vi "IntelligentServo.vi"(2 "timeout (s) 2":dbl=10.0 caption="ONTime" format="%0.2f", 3 "number of samples":i32=30, 4 "timeout (s)":dbl=10.0 format="%0.2f", 5 "error in":errorcluster, 7 "stop (T)":bool=TRUE, 10 "device name":tag="myDAQ1") -> (14 "task out":refnum<k21>, 19 "error out":errorcluster)   [LabVIEW 2023]
doc: "Creates, edits, and runs tasks using NI-DAQmx. Refer to the NI-DAQmx Readme for a complete listing of devices NI-DAQmx supports.\n\nWhen you place this Express VI on the block diagram, the DAQ Assistant launches to create a new task. After you create a task, you can double-click the DAQ Assistant Express VI to edit that task. For continuous measurement or generation, place a while loop around the DAQ Assistant Express VI.\n\nUsing the DAQ Assistant Express VI creates a task accessible only to the Express VI. To make the task globally accessible from any application, you must convert the Express VI to an NI-DAQmx task saved in MAX\n\nYou can generate NI-DAQmx API code from a DAQ Assistant Express VI. Right-click the DAQ Assistant Express VI and select <B> Generate NI-DAQmx Code</B> from the shortcut menu to generate both configuration and example code for the task.\n\nFor continuous single-point input or output, the DAQ Assistant Express VI might not provide optimal performance. Refer to the Cont Acq&Graph Voltage-Single Point Optimization VI in examples\\DAQmx\\Analog In\\Measure Voltage.llb for an example of techniques to create higher-performance, single-point I/O applications."
uses:
  <vilib>/DAQmx/create/channels.llb/DAQmx Create Channel (CO-Pulse Generation-Time).vi
  <vilib>/DAQmx/configure/timing.llb/DAQmx Timing (Implicit).vi
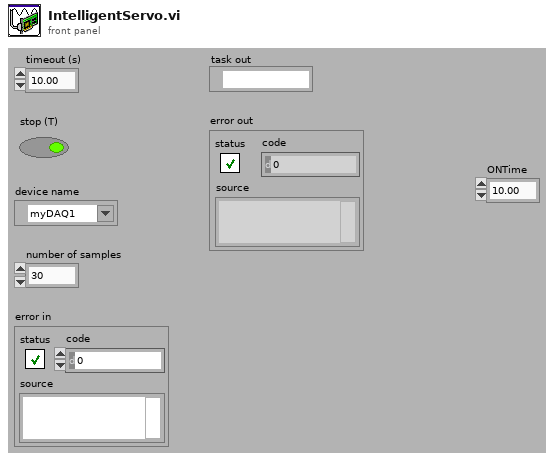
[diagram p1: front panel]
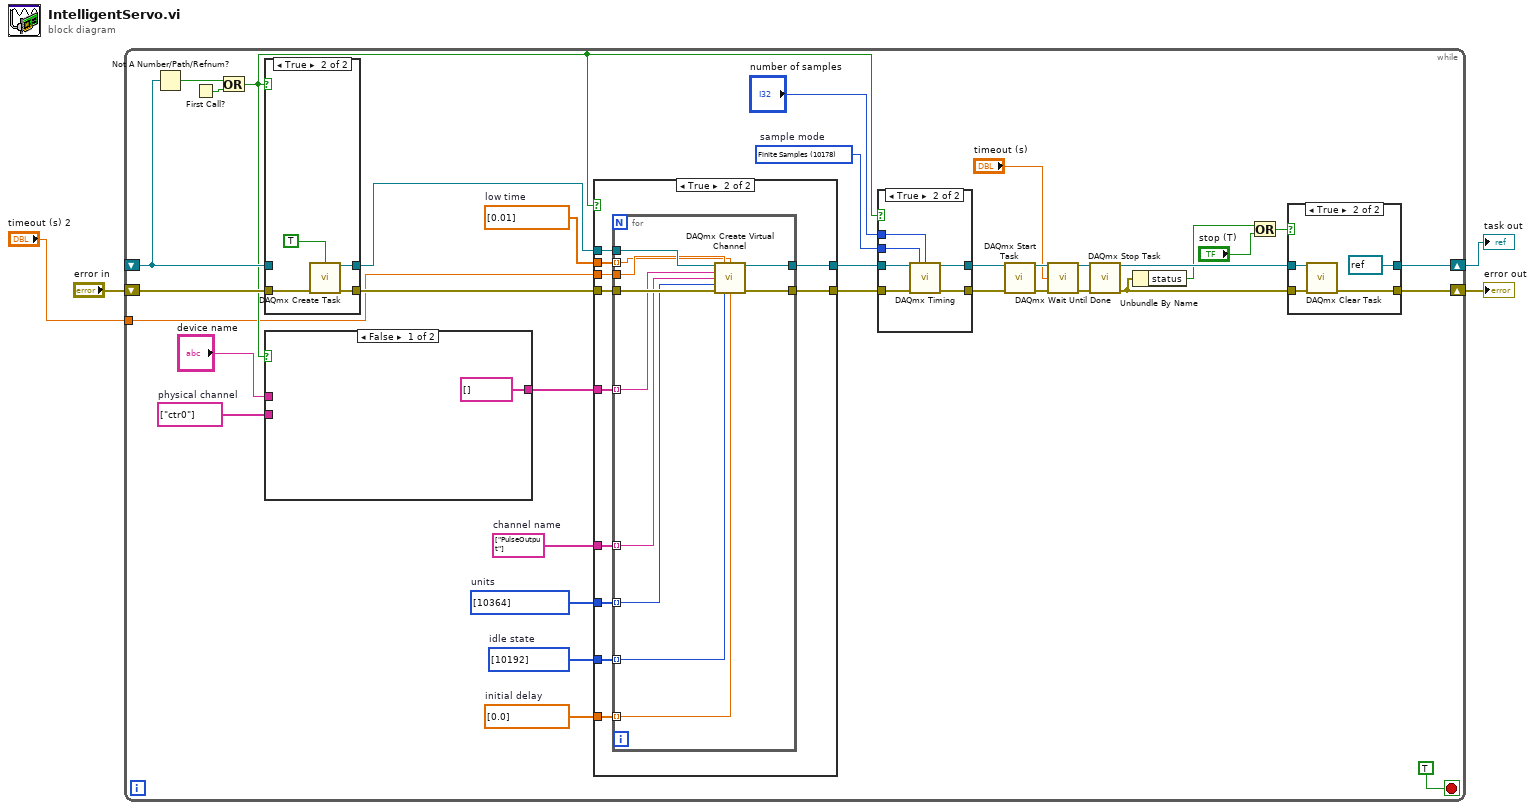
[diagram p0: block diagram]
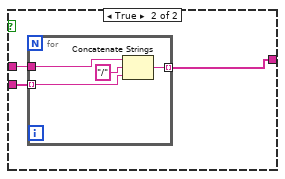
[diagram p5: hidden frame]
diagram:
  n1 = while {
    shift-right: [w12] -> w2
    shift-left: _ -> [w36]
    shift-right: [w6] -> w3
    shift-left: "error in" -> [w37]
    tunnel: "timeout (s) 2" -> [w5]
    stop <- TRUE stop-if-true
    w20 = 10178 items=["Finite Samples"=10178, "Continuous Samples"=10123, "Hardware Timed Single Point"=12522]  # sample mode
    w25 = dbl[] [0.0]  # initial delay
    w26 = i32[] [10192] items=["High"=10192, "Low"=10214]  # idle state
    w27 = i32[] [10364] items=["Seconds"=10364, "From Custom Scale"=10065]  # units
    w28 = string[] ["PulseOutput"]  # channel name
    w30 = dbl[] [0.01]  # low time
    w33 = string[] ["ctr0"]  # physical channel
    n2 = Not A Number/Path/Refnum?(number/path/refnum=w36) -> (NaN/Path/Refnum?=w35:bool)
    n3 = First Call?() -> (First Call?: T/F=w38:bool)
    n4 = Or(x=w35, y=w38) -> (x .or. y?=w24:bool)
    n5 = case shown="True" w24 {
      tunnel: [w87 w91] -> w32
      tunnel: w36 -> [w87 _]
      tunnel: [w86 w90] -> w31
      tunnel: w37 -> [w86 w88]
      frame False {
      }
      frame True {
        n6 = call <vilib>:"DAQmx Create Task.vi"("auto cleanup"=TRUE, "error in"=w88) -> ("task out"=w91:refnum<k21>, "error out"=w90:errorcluster)  [unwired: 12 in]
      }
    }
    n7 = case shown="False" w24 {
      tunnel: [string[] [] w81] -> w29
      tunnel: "device name" -> [_ w80]
      tunnel: w33 -> [_ w79]
      frame False {
      }
      frame True {
        n8 = for {
          tunnel: [w85] -> w81 mode=indexing
          tunnel: w80 -> [w84]
          tunnel: w79 -> [w82] mode=indexing
          n9 = Concatenate Strings(w84, "/" ("string"), w82) -> (w85:string)
        }
      }
    }
    n10 = case shown="True" w24 {
      tunnel: [w55 w66] -> w23
      tunnel: w32 -> [w55 w65]
      tunnel: [w54 w64] -> w22
      tunnel: w31 -> [w54 w63]
      tunnel: w30 -> [_ w62]
      tunnel: w5 -> [_ w61]
      tunnel: w29 -> [_ w60]
      tunnel: w28 -> [_ w59]
      tunnel: w27 -> [_ w58]
      tunnel: w26 -> [_ w57]
      tunnel: w25 -> [_ w56]
      frame False {
      }
      frame True {
        n11 = for {
          tunnel: [w77] -> w66
          tunnel: w65 -> [w76]
          tunnel: [w75] -> w64
          tunnel: w63 -> [w74]
          tunnel: w60 -> [w73] mode=indexing
          tunnel: w61 -> [w72]
          tunnel: w62 -> [w71] mode=indexing
          tunnel: w59 -> [w70] mode=indexing
          tunnel: w58 -> [w69] mode=indexing
          tunnel: w57 -> [w68] mode=indexing
          tunnel: w56 -> [w67] mode=indexing
          n12 = call-poly <vilib>:"DAQmx Create Virtual Channel.vi"("task in"=w76, "high time"=w72, "low time"=w71, "counter"=w73, "name to assign"=w70, "units"=w69, "error in"=w74, "idle state"=w68, "initial delay"=w67) -> ("task out"=w77:refnum<k21>, "error out"=w75:errorcluster)  [unwired: 5 in]
        }
      }
    }
    n13 = case shown="True" w24 {
      tunnel: [w47 w51] -> w15
      tunnel: w23 -> [w47 w53]
      tunnel: [w46 w50] -> w14
      tunnel: w22 -> [w46 w52]
      tunnel: w20 -> [_ w49]
      tunnel: "number of samples" -> [_ w48]
      frame False {
      }
      frame True {
        n14 = call-poly <vilib>:"DAQmx Timing.vi"("task/channels in"=w53, "sample mode"=w49, "samples per channel"=w48, "error in"=w52) -> ("task out"=w51:refnum<k21>, "error out"=w50:errorcluster)  [unwired: 10 in]
      }
    }
    n15 = call <vilib>:"DAQmx Start Task.vi"("task/channels in"=w15, "error in"=w14) -> ("task out"=w19:refnum<k21>, "error out"=w18:errorcluster)  [unwired: 12 in]
    n16 = call <vilib>:"DAQmx Wait Until Done.vi"("task/channels in"=w19, "timeout (sec)"="timeout (s)", "error in"=w18) -> ("task out"=w16:refnum<k21>, "error out"=w17:errorcluster)  [unwired: 11 in]
    n17 = call <vilib>:"DAQmx Stop Task.vi"("task/channels in"=w16, "error in"=w17) -> ("task out"=w13:refnum<k21>, "error out"=w10:errorcluster)  [unwired: 12 in]
    n18 = Unbundle By Name(w10) -> ("status"=w9:bool)
    n19 = Or(x=w9, y="stop (T)") -> (x .or. y?=w7:bool)
    n20 = case shown="True" w7 {
      tunnel: w13 -> [w41 w45]
      tunnel: [w41 refnum<k21> refnum ("task in")] -> w12
      tunnel: w10 -> [w40 w44]
      tunnel: [w40 w43] -> w6
      frame False {
      }
      frame True {
        n21 = call <vilib>:"DAQmx Clear Task.vi"("task in"=w45, "error in"=w44) -> ("error out"=w43:errorcluster)  [unwired: 13 in]
      }
    }
  }
  "error out" <- w3
  "task out" <- w2
